vi "AMC Multiple Targets Example 1.vi"() -> ()   [LabVIEW 2009]
uses:
  <vilib>/NI/Tools/Keyed Array/KeyedArray.ctl
  vi.lib/NI/AMC/AMC.lvlib
  <vilib>/NI/Tools/Keyed Array/Tools_KeyedArray.lvlib
panel:
  in  "Local UDP Port":u16=8000
  in  "Target UDP Port":u16=9000
  in  "Servers":i32(listbox)
  in  "Get All Queues":bool
  in  "Target IP Address":string="10.0.18.197"
  in  "Queue":string
  in  "Verify Queue":bool
  in  "PingAll":bool
  out "Response":string
  in  "Ping":bool
  in  "Remote Exit":bool
  out "Process":bool
  in  "Remote Process":bool
  out "Status":string
  in  "Local Process":bool
  in  "Local Exit":bool
  in  "State Variables":T1
  # "Target 1"
  # "Local Messages >>"
  # "Remote Messages >>"
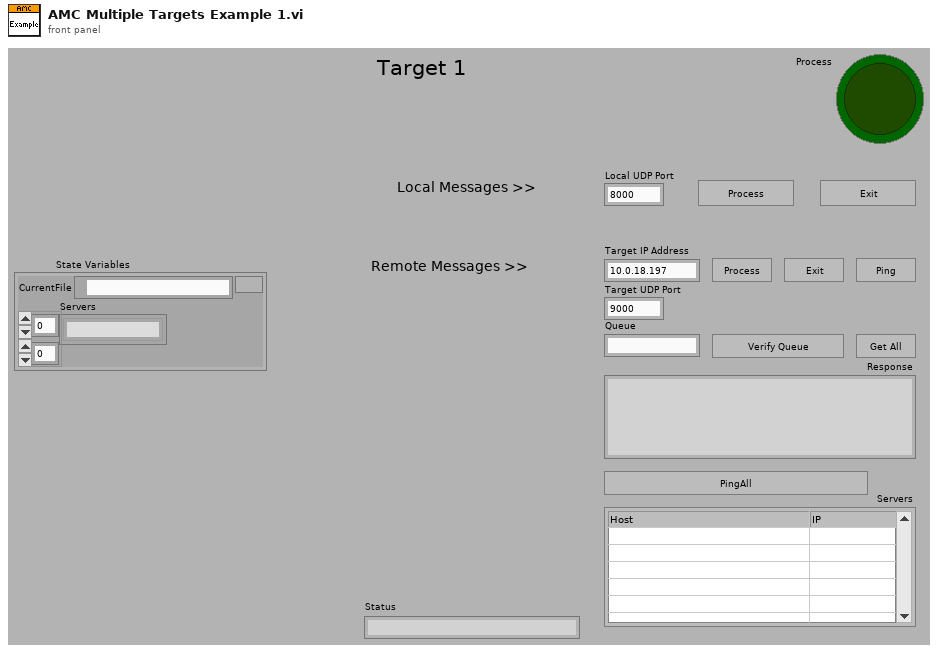
[diagram p1: front panel]
types:
  T1 = cluster{"CurrentFile":path, "Servers":string[][]}
  T2 = typedef "AMC.lvlib/Message Queue.ctl" = refnum<queue>
  T3 = typedef "Tools_KeyedArray.lvlib/KeyedArray.ctl" = cluster{"keys":string[], "values":string[]}
  T4 = typedef "LVPoint32TypeDef.ctl" = cluster{"Horizontal":i32, "Vertical":i32}
  T5 = typedef "LVRowAndColumnTypeDef.ctl" = cluster{"Row":i32, "Column":i32}
  T6 = typedef "AMC.lvlib/Message.ctl" = cluster{"name":string, "value":string, "attributes":T3, "receiver host":string, "receiver process":string, "source host":string, "source process":string, "priority message":bool, "acknowledge message":bool}
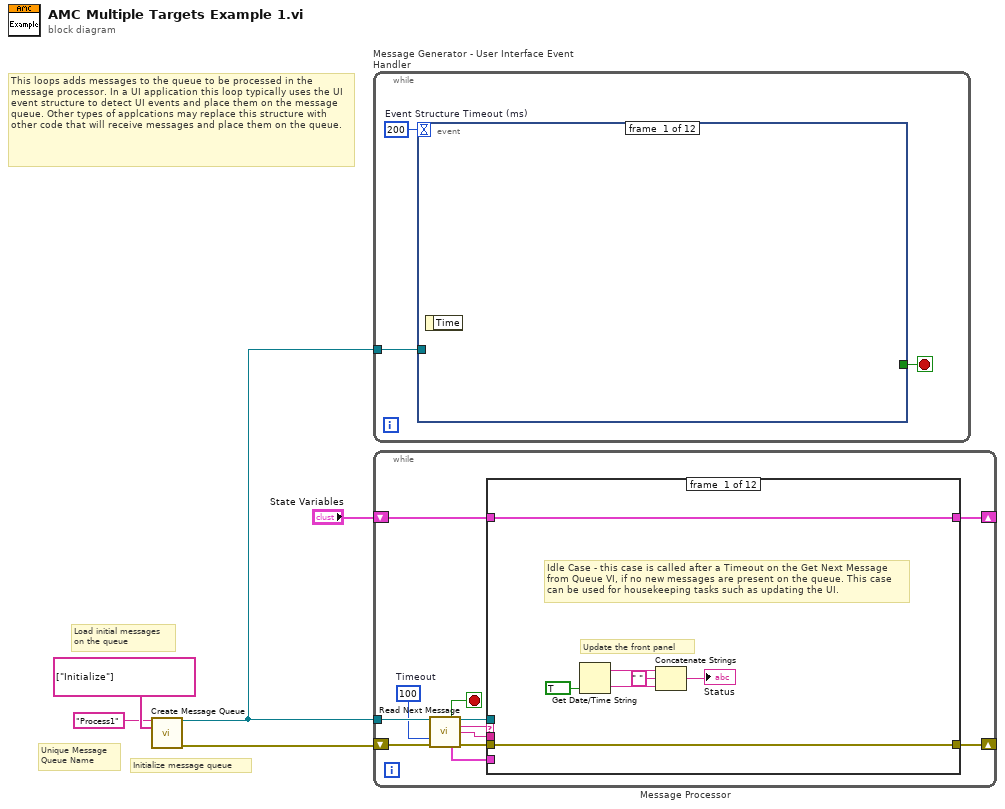
[diagram p0: block diagram]
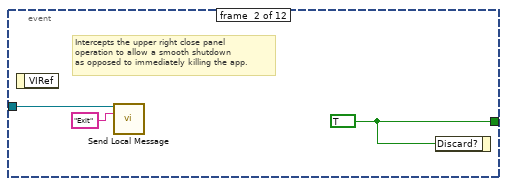
[diagram p2: hidden frame]
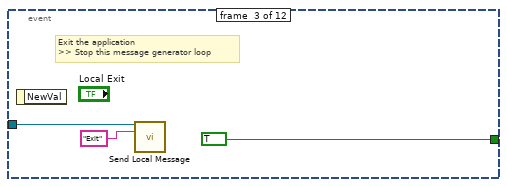
[diagram p3: hidden frame]
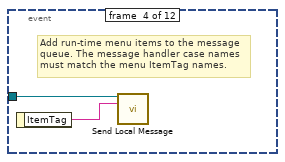
[diagram p4: hidden frame]
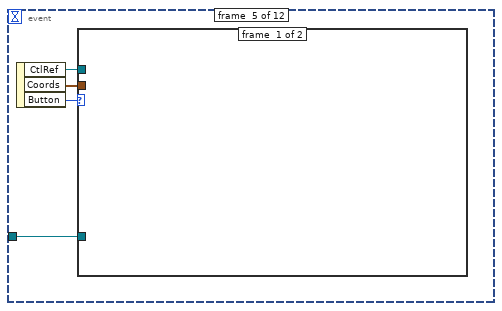
[diagram p5: hidden frame]
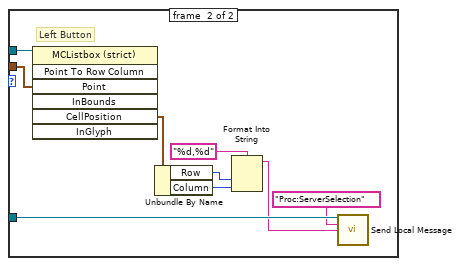
[diagram p6: hidden frame]
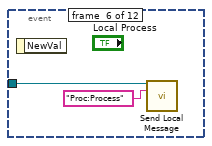
[diagram p7: hidden frame]
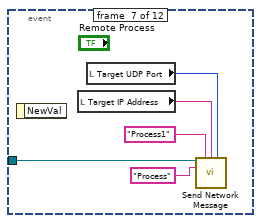
[diagram p8: hidden frame]
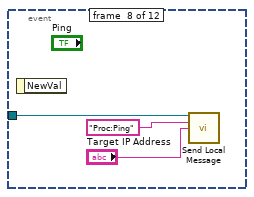
[diagram p9: hidden frame]
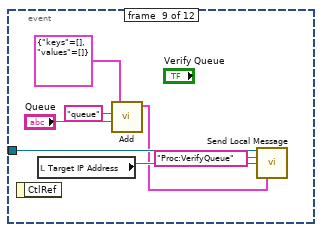
[diagram p10: hidden frame]
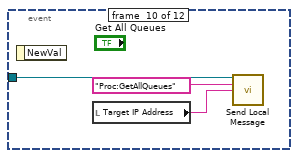
[diagram p11: hidden frame]
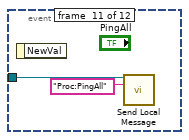
[diagram p12: hidden frame]
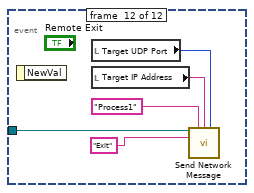
[diagram p13: hidden frame]
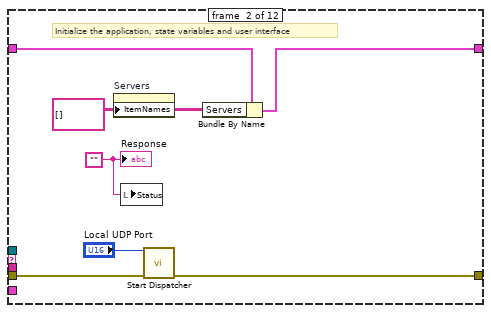
[diagram p14: hidden frame]
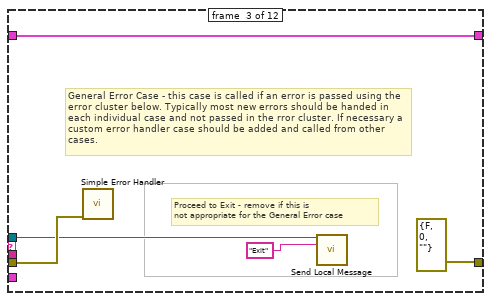
[diagram p15: hidden frame]
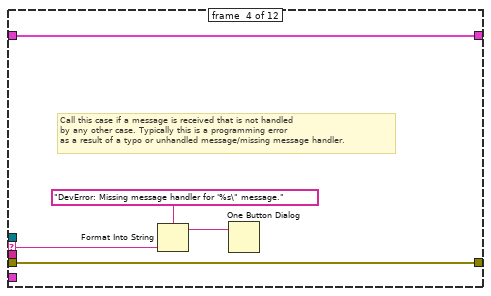
[diagram p16: hidden frame]
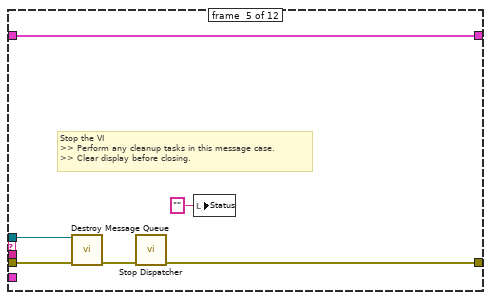
[diagram p17: hidden frame]
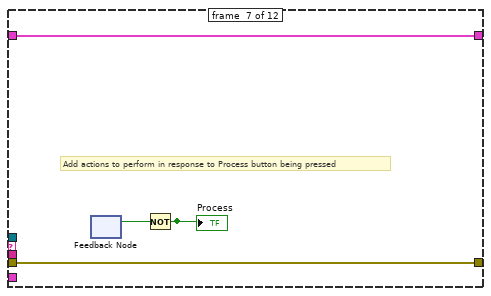
[diagram p19: hidden frame]
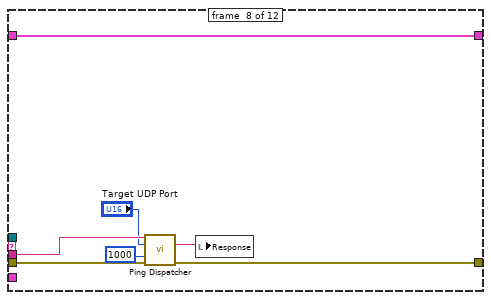
[diagram p20: hidden frame]
diagram:
  # "This loops adds messages to the queue to be processed in the message processor. In a UI application this loop typically uses the UI event structure to detect UI events and place them on the message queue. Other types of applcations may replace this structure with other code that will receive messages and place them on the queue."
  # "Initialize message queue"
  # "Unique Message\nQueue Name"
  # "Load initial messages\non the queue"
  n1 = call "Create Message Queue.vi"("message queue name"="Process1" ("Message queue name (unnamed)"), "initial message names"=string[] ["Initialize"]) -> ("message queue out"=w5:T2, "error out"=w3:errorcluster)  [unwired: 12 in]
  n2 = while "Message Generator - User Interface Event Handler" {
    tunnel: w5 -> [w6]
    stop <- w7 stop-if-true
    w8 = 200  # Event Structure Timeout (ms)
    n3 = event shown="[11] \"Remote Exit\": Value Change" {
      selector: _ -> [_ _ _ _ _ _ _ _ _ _ _ _]
      dyn-events: _ -> [_ _ _ _ _ _ _ _ _ _ _ _]
      timeout: w8 -> [_ _ _ _ _ _ _ _ _ _ _ _]
      tunnel: [_ w11 TRUE ("Discard?") _ _ _ _ _ _ _ _ _] -> w7
      tunnel: w6 -> [_ w9 w13 w15 w20 w31 w36 w39 w46 w49 w51 w56]
      event #0 {
        n4 = event-data() -> ()  [unwired: 2 out]
      }
      event #1 {
        w11 = TRUE ("Discard?")
        # "Intercepts the upper right close panel\noperation to allow a smooth shutdown\nas opposed to immediately killing the app."
        n5 = event-data() -> ()  [unwired: 2 out]
        n6 = call "Send Local Message.vi"("message queue in"=w9, "message name"="Exit") -> ()  [unwired: 11 in, 3 out]
        n7 = event-data("Discard?"=w11) -> ()  [unwired: 1 in, 1 out]
      }
      event #2 {
        # "Exit the application\n>> Stop this message generator loop"
        n8 = event-data() -> ()  [unwired: 2 out]
        n9 = call "Send Local Message.vi"("message queue in"=w13, "message name"="Exit") -> ()  [unwired: 11 in, 3 out]
      }
      event #3 {
        # "Add run-time menu items to the message\nqueue. The message handler case names must match the menu ItemTag names."
        n10 = event-data() -> ("ItemTag"=w16:string)  [unwired: 1 out]
        n11 = call "Send Local Message.vi"("message queue in"=w15, "message name"=w16) -> ()  [unwired: 11 in, 3 out]
      }
      event #4 {
        n12 = event-data() -> ("CtlRef"=w19:refnum<vi>, "Coords"=w18:T4, "Button"=w17:u16)  [unwired: 1 out]
        n13 = case shown="1" w17 {
          tunnel: w20 -> [_ w29]
          tunnel: w19 -> [_ w27]
          tunnel: w18 -> [_ w26]
          frame #0 {
          }
          frame #1 {
            # "Left Button"
            n14 = invoke class="MCListbox (strict)" method="Point To Row Column"(reference=w27, "Point"=w26) -> ("CellPosition"=w25:T5)  [unwired: 5 in, 6 out]
            n15 = Unbundle By Name(w25) -> ("Row"=w24:i32, "Column"=w23:i32)
            n16 = Format Into String(format string="%d,%d", w24, w23) -> (resulting string=w21:string)  [unwired: 2 in, 1 out]
            n17 = call "Send Local Message.vi"("message queue in"=w29, "message name"="Proc:ServerSelection" ("Message Name"), "message value"=w21) -> ()  [unwired: 10 in, 3 out]
          }
        }
      }
      event #5 {
        n18 = event-data() -> ()  [unwired: 2 out]
        n19 = call "Send Local Message.vi"("message queue in"=w31, "message name"="Proc:Process") -> ()  [unwired: 11 in, 3 out]
      }
      event #6 {
        n20 = event-data() -> ()  [unwired: 2 out]
        n21 = local read "Target IP Address"() -> (w33:string)
        n22 = local read "Target UDP Port"() -> (w32:u16)
        n23 = call "Send Network Message.vi"("message queue in"=w36, "receiver process"="Process1" ("process"), "receiver host"=w33, "receiver port (0)"=w32, "message name"="Process") -> ()  [unwired: 8 in, 3 out]
      }
      event #7 {
        n24 = event-data() -> ()  [unwired: 2 out]
        n25 = call "Send Local Message.vi"("message queue in"=w39, "message name"="Proc:Ping" ("Message Name"), "message value"="Target IP Address") -> ()  [unwired: 10 in, 3 out]
      }
      event #8 {
        n26 = event-data() -> ()  [unwired: 2 out]
        n27 = local read "Target IP Address"() -> (w44:string)
        n28 = call <vilib>:"Add.vi"("value"="Queue", "key"="queue", "array in"=T3 {"keys"=[], "values"=[]}) -> ("array out"=w40:T3)  [unwired: 1 in, 3 out]
        n29 = call "Send Local Message.vi"("message queue in"=w46, "message name"="Proc:VerifyQueue" ("Message Name"), "message value"=w44, "message attributes"=w40) -> ()  [unwired: 9 in, 3 out]
      }
      event #9 {
        n30 = event-data() -> ()  [unwired: 2 out]
        n31 = local read "Target IP Address"() -> (w47:string)
        n32 = call "Send Local Message.vi"("message queue in"=w49, "message name"="Proc:GetAllQueues" ("Message Name"), "message value"=w47) -> ()  [unwired: 10 in, 3 out]
      }
      event #10 {
        n33 = event-data() -> ()  [unwired: 2 out]
        n34 = call "Send Local Message.vi"("message queue in"=w51, "message name"="Proc:PingAll" ("Message Name")) -> ()  [unwired: 11 in, 3 out]
      }
      event #11 {
        n35 = event-data() -> ()  [unwired: 2 out]
        n36 = local read "Target UDP Port"() -> (w52:u16)
        n37 = local read "Target IP Address"() -> (w53:string)
        n38 = call "Send Network Message.vi"("message queue in"=w56, "receiver process"="Process1" ("process"), "receiver host"=w53, "receiver port (0)"=w52, "message name"="Exit") -> ()  [unwired: 8 in, 3 out]
      }
    }
  }
  n39 = while "Message Processor" {
    shift-left: w3 -> [w63]
    shift-right: [w64] -> _
    tunnel: w5 -> [w62]
    shift-left: "State Variables" -> [w68]
    shift-right: [w67] -> _
    stop <- w61 stop-if-true
    w57 = 100  # Timeout
    n40 = call "Read Next Message.vi"("message queue in"=w62, "timeout (1 ms)"=w57, "error in"=w63) -> ("exit process?"=w61:bool, "message queue out"=w66:T2, "message name"=w60:string, "message value"=w59:string, "message"=w58:T6, "error out"=w65:errorcluster)  [unwired: 5 in, 2 out]
    n41 = case shown="\"Proc:GetAllQueues\"" w60 {
      selector: w60 -> [_ _ _ w90 _ _ _ _ _ _ _ _]
      tunnel: [w75 w78 w87 w92 w97 w100 w103 w111 w114 w137 w143 w151] -> w67
      tunnel: w68 -> [w75 w79 w87 w92 w97 w100 w103 w111 w115 w137 w143 w151]
      tunnel: w66 -> [_ _ w84 _ w95 _ _ _ _ _ _ _]
      tunnel: w65 -> [w74 w81 w85 w91 w98 w99 w104 w110 w120 w131 w140 w150]
      tunnel: [w74 w80 errorcluster {"status"=FALSE, "code"=0, "source"=""} ("error out") w91 w93 w99 w104 w109 w119 w130 w139 w150] -> w64
      tunnel: w58 -> [_ _ _ _ _ _ _ _ _ w136 _ _]
      tunnel: w59 -> [_ _ _ _ _ _ _ w107 _ w133 w142 w147]
      frame #0 {
        # "Update the front panel"
        # "Idle Case - this case is called after a Timeout on the Get Next Message from Queue VI, if no new messages are present on the queue. This case can be used for housekeeping tasks such as updating the UI."
        n42 = Get Date/Time String(want seconds? (F)=TRUE) -> (date string=w73:string, time string=w72:string)  [unwired: 2 out]
        n43 = Concatenate Strings(w73, " " ("string"), w72) -> (→"Status":string)
      }
      frame #1 {
        w77 = string[][] [] ("Item Names")
        w82 = ""
        # "Initialize the application, state variables and user interface"
        n44 = property on="Servers" class="MCListbox (strict)"("ItemNames"=w77) -> ()  [unwired: 2 in, 2 out]
        n45 = local write "Status"(w82) -> ()
        n46 = call "Start Dispatcher.vi"("UDP port (0)"="Local UDP Port", "error in"=w81) -> ("error out"=w80:errorcluster)  [unwired: 11 in, 2 out]
        n47 = Bundle By Name(cluster=w79, "Servers"=w77) -> (w78:T1)
        "Response" <- w82
      }
      frame #2 {
        # "Proceed to Exit - remove if this is\nnot appropriate for the General Error case"
        # "General Error Case - this case is called if an error is passed using the error cluster below. Typically most new errors should be handed in each individual case and not passed in the rror cluster. If necessary a custom error handler case should be added and called from other cases."
        n48 = call <vilib>:"Simple Error Handler.vi"("error in (no error)"=w85) -> ()  [unwired: 1 in, 8 out]
        n49 = call "Send Local Message.vi"("message queue in"=w84, "message name"="Exit") -> ()  [unwired: 11 in, 3 out]
      }
      frame #3 {
        # "Call this case if a message is received that is not handled \nby any other case. Typically this is a programming error\nas a result of a typo or unhandled message/missing message handler."
        n50 = Format Into String(format string="DevError: Missing message handler for '%s\" message." ("message"), w90) -> (resulting string=w88:string)  [unwired: 2 in, 1 out]
        n51 = One Button Dialog(message=w88) -> ()  [unwired: 2 out]
      }
      frame #4 {
        # "Stop the VI\n>> Perform any cleanup tasks in this message case.\n>> Clear display before closing."
        n52 = call "Destroy Message Queue.vi"("message queue in"=w95, "error in"=w98) -> ("error out"=w94:errorcluster)  [unwired: 11 in, 2 out]
        n53 = call "Stop Dispatcher.vi"("error in"=w94) -> ("error out"=w93:errorcluster)  [unwired: 14 in]
        n54 = local write "Status"("" ("Status")) -> ()
      }
      frame #5 {
      }
      frame #6 {
        # "Add actions to perform in response to Process button being pressed"
        n55 = feedback #1() -> (w102:bool)  [unwired: 1 out]
        n56 = Not(x=w102) -> (.not. x?=w101:bool)
        "Process" <- w101
      }
      frame #7 {
        n57 = call "Ping Dispatcher.vi"("receiver host (\"\")"=w107, "receiver port (0)"="Target UDP Port", "timeout (100 ms)"=1000 ("Timeout (100 ms)"), "error in"=w110) -> ("string response"=w108:string, "error out"=w109:errorcluster)  [unwired: 9 in, 1 out]
        n58 = local write "Response"(w108) -> ()
      }
      frame #8 {
        n59 = local read "Target UDP Port"() -> (w112:u16)
        n60 = call "Ping All Dispatchers.vi"("receiver port (0)"=w112, "timeout (1000 ms)"=1000 ("Timeout (1000 ms)"), "error in"=w120) -> ("response messages"=w116:T6[], "response"=w118:string, "error out"=w119:errorcluster)  [unwired: 10 in]
        n61 = for {
          tunnel: w116 -> [w126] mode=indexing
          tunnel: [w121] -> w113 mode=indexing
          n62 = Unbundle By Name(w126) -> ("source host"=w123:string, "attributes"=w125:T3)
          n63 = call <vilib>:"Index.vi"("key"="IP", "array in"=w125) -> ("value"=w122:string)  [unwired: 2 in, 3 out]
          n64 = Build Array(w123, w122) -> (w121:string[])
        }
        n65 = local write "Response"(w118) -> ()
        n66 = property on="Servers" class="MCListbox (strict)"("ItemNames"=w113) -> ()  [unwired: 2 in, 2 out]
        n67 = Bundle By Name(cluster=w115, "Servers"=w113) -> (w114:T1)
      }
      frame #9 {
        n68 = Unbundle By Name(w136) -> ("attributes"=w135:T3)
        n69 = call <vilib>:"Index.vi"("key"="queue", "array in"=w135) -> ("value"=w128:string)  [unwired: 2 in, 3 out]
        n70 = local read "Target UDP Port"() -> (w127:u16)
        n71 = call "Verify Dispatcher Queue.vi"("receiver host (\"\")"=w133, "receiver port (0)"=w127, "queue name"=w128, "timeout (100 ms)"=1000 ("Timeout (100 ms)"), "error in"=w131) -> ("string response"=w132:string, "error out"=w130:errorcluster)  [unwired: 8 in, 1 out]
        n72 = local write "Response"(w132) -> ()
      }
      frame #10 {
        n73 = local read "Target UDP Port"() -> (w138:u16)
        n74 = call "Get All Dispatcher Queues.vi"("receiver host (\"\")"=w142, "receiver port (0)"=w138, "error in"=w140) -> ("string response"=w141:string, "error out"=w139:errorcluster)  [unwired: 9 in, 2 out]
        n75 = local write "Response"(w141) -> ()
      }
      frame #11 {
        n76 = Unbundle By Name(w151) -> ("Servers"=w149:string[][])
        n77 = Scan From String(format string="%d,%d", input string=w147) -> (output 1=w145:i32, output 2=w144:i32)  [unwired: 2 in, 5 out]
        n78 = Index Array(array=w149, index (row)=w145, index (col)=w144) -> (element=w148:string)
        n79 = local write "Target IP Address"(w148) -> ()
      }
    }
  }
